vi "CHECK BATT DATA.vi"(10 "DATA":dbl[](array[numeric]), 11 "BATTERY EMULATOR":T1) -> (3 "result":bool)   [LabVIEW 2018]
panel:
  out "POWER":bool
  out "CURRENT":bool
  out "VOLTAGE":bool
  out "CONTROL SELECTED":bool
  out "MODE SELECTED":bool
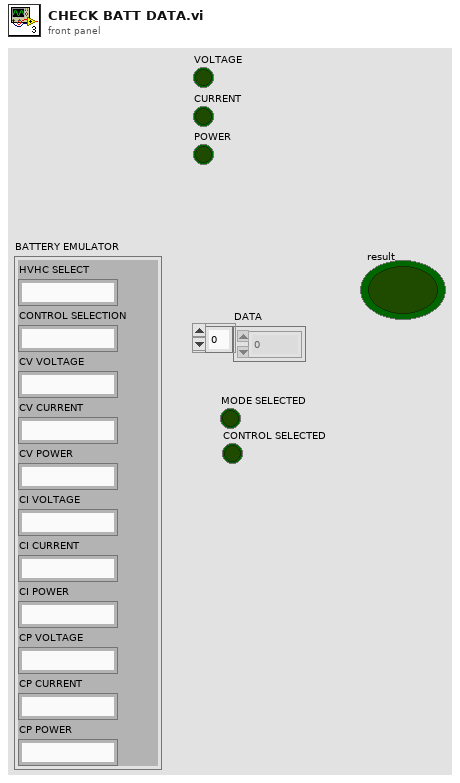
[diagram p1: front panel]
types:
  T1 = cluster{"HVHC SELECT":string, "CONTROL SELECTION":string, "CV VOLTAGE":string, "CV CURRENT":string, "CV POWER":string, "CI VOLTAGE":string, "CI CURRENT":string, "CI POWER":string, "CP VOLTAGE":string, "CP CURRENT":string, "CP POWER":string}
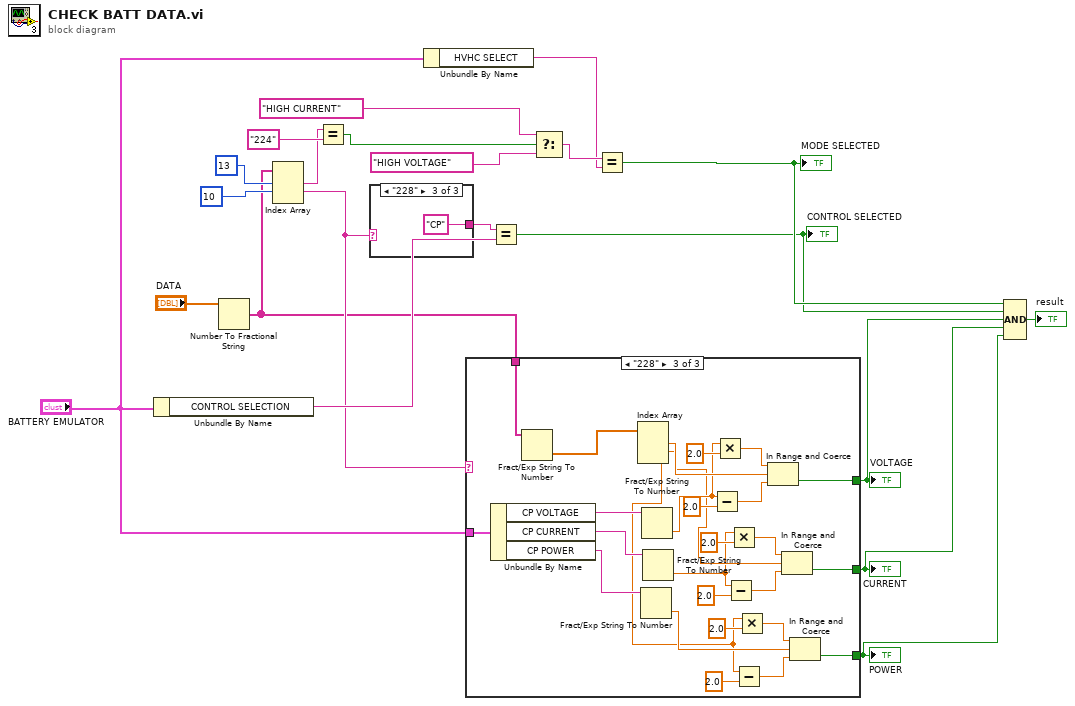
[diagram p0: block diagram]
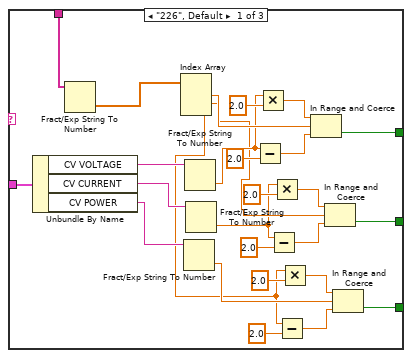
[diagram p2: hidden frame]
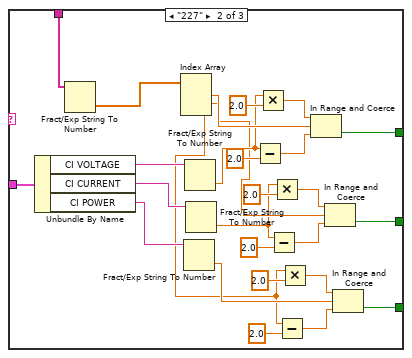
[diagram p3: hidden frame]
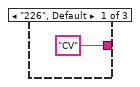
[diagram p4: hidden frame]
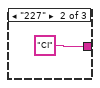
[diagram p5: hidden frame]
diagram:
  n1 = Unbundle By Name("BATTERY EMULATOR") -> ("CONTROL SELECTION"=w10:string)
  n2 = Number To Fractional String(number="DATA") -> (F-format string=w7:string[])  [unwired: 3 in]
  n3 = Index Array(array=w7, index #1=13 ("index"), index #2=10 ("index")) -> (element #1=w11:string, element #2=w9:string)  [unwired: 1 in, 1 out]
  n4 = Equal?(x=w11, y="224") -> (x = y?=w18:bool)
  n5 = case shown="\"228\"" w9 {
    tunnel: ["CV" "CI" "CP"] -> w12
    frame "226", Default {
    }
    frame "227" {
    }
    frame "228" {
    }
  }
  n6 = Unbundle By Name("BATTERY EMULATOR") -> ("HVHC SELECT"=w13:string)
  n7 = case shown="\"228\"" w9 {
    tunnel: "BATTERY EMULATOR" -> [w51 w78 w105]
    tunnel: w7 -> [w50 w77 w104]
    tunnel: [w39 w66 w93] -> w4
    tunnel: [w32 w59 w86] -> w3
    tunnel: [w26 w53 w80] -> w2
    frame "226", Default {
      n8 = Unbundle By Name(w51) -> ("CV VOLTAGE"=w48:string, "CV CURRENT"=w47:string, "CV POWER"=w46:string)
      n9 = Fract/Exp String To Number(string=w50) -> (number=w49:dbl[])  [unwired: 3 in, 1 out]
      n10 = Index Array(array=w49) -> (element #1=w45:dbl, element #2=w34:dbl, element #3=w25:dbl)  [unwired: 3 in]
      n11 = Fract/Exp String To Number(string=w46) -> (number=w27:dbl)  [unwired: 3 in, 1 out]
      n12 = Fract/Exp String To Number(string=w48) -> (number=w40:dbl)  [unwired: 3 in, 1 out]
      n13 = Fract/Exp String To Number(string=w47) -> (number=w33:dbl)  [unwired: 3 in, 1 out]
      n14 = Subtract(x=w40, y=2.0) -> (x-y=w43:dbl)
      n15 = Multiply(x=w40, y=2.0) -> (x*y=w41:dbl)
      n16 = Subtract(x=w33, y=2.0) -> (x-y=w36:dbl)
      n17 = Multiply(x=w33, y=2.0) -> (x*y=w38:dbl)
      n18 = Subtract(x=w25, y=2.0) -> (x-y=w30:dbl)
      n19 = Multiply(x=w25, y=2.0) -> (x*y=w28:dbl)
      n20 = In Range and Coerce(upper limit=w41, x=w45, lower limit=w43) -> (In Range?=w39:bool)  [unwired: 1 out]
      n21 = In Range and Coerce(upper limit=w38, x=w34, lower limit=w36) -> (In Range?=w32:bool)  [unwired: 1 out]
      n22 = In Range and Coerce(upper limit=w28, x=w27, lower limit=w30) -> (In Range?=w26:bool)  [unwired: 1 out]
    }
    frame "227" {
      n23 = Unbundle By Name(w78) -> ("CI VOLTAGE"=w75:string, "CI CURRENT"=w74:string, "CI POWER"=w73:string)
      n24 = Fract/Exp String To Number(string=w77) -> (number=w76:dbl[])  [unwired: 3 in, 1 out]
      n25 = Index Array(array=w76) -> (element #1=w72:dbl, element #2=w61:dbl, element #3=w52:dbl)  [unwired: 3 in]
      n26 = Fract/Exp String To Number(string=w73) -> (number=w54:dbl)  [unwired: 3 in, 1 out]
      n27 = Fract/Exp String To Number(string=w75) -> (number=w67:dbl)  [unwired: 3 in, 1 out]
      n28 = Fract/Exp String To Number(string=w74) -> (number=w60:dbl)  [unwired: 3 in, 1 out]
      n29 = Subtract(x=w67, y=2.0) -> (x-y=w70:dbl)
      n30 = Multiply(x=w67, y=2.0) -> (x*y=w68:dbl)
      n31 = Subtract(x=w60, y=2.0) -> (x-y=w63:dbl)
      n32 = Multiply(x=w60, y=2.0) -> (x*y=w65:dbl)
      n33 = Subtract(x=w52, y=2.0) -> (x-y=w57:dbl)
      n34 = Multiply(x=w52, y=2.0) -> (x*y=w55:dbl)
      n35 = In Range and Coerce(upper limit=w68, x=w72, lower limit=w70) -> (In Range?=w66:bool)  [unwired: 1 out]
      n36 = In Range and Coerce(upper limit=w65, x=w61, lower limit=w63) -> (In Range?=w59:bool)  [unwired: 1 out]
      n37 = In Range and Coerce(upper limit=w55, x=w54, lower limit=w57) -> (In Range?=w53:bool)  [unwired: 1 out]
    }
    frame "228" {
      n38 = Unbundle By Name(w105) -> ("CP VOLTAGE"=w102:string, "CP CURRENT"=w101:string, "CP POWER"=w100:string)
      n39 = Fract/Exp String To Number(string=w104) -> (number=w103:dbl[])  [unwired: 3 in, 1 out]
      n40 = Index Array(array=w103) -> (element #1=w99:dbl, element #2=w88:dbl, element #3=w79:dbl)  [unwired: 3 in]
      n41 = Fract/Exp String To Number(string=w100) -> (number=w81:dbl)  [unwired: 3 in, 1 out]
      n42 = Fract/Exp String To Number(string=w102) -> (number=w94:dbl)  [unwired: 3 in, 1 out]
      n43 = Fract/Exp String To Number(string=w101) -> (number=w87:dbl)  [unwired: 3 in, 1 out]
      n44 = Subtract(x=w94, y=2.0) -> (x-y=w97:dbl)
      n45 = Multiply(x=w94, y=2.0) -> (x*y=w95:dbl)
      n46 = Subtract(x=w87, y=2.0) -> (x-y=w90:dbl)
      n47 = Multiply(x=w87, y=2.0) -> (x*y=w92:dbl)
      n48 = Subtract(x=w79, y=2.0) -> (x-y=w84:dbl)
      n49 = Multiply(x=w79, y=2.0) -> (x*y=w82:dbl)
      n50 = In Range and Coerce(upper limit=w95, x=w99, lower limit=w97) -> (In Range?=w93:bool)  [unwired: 1 out]
      n51 = In Range and Coerce(upper limit=w92, x=w88, lower limit=w90) -> (In Range?=w86:bool)  [unwired: 1 out]
      n52 = In Range and Coerce(upper limit=w82, x=w81, lower limit=w84) -> (In Range?=w80:bool)  [unwired: 1 out]
    }
  }
  "VOLTAGE" <- w4
  "CURRENT" <- w3
  "POWER" <- w2
  n53 = Equal?(x=w12, y=w10) -> (x = y?=w5:bool)
  "CONTROL SELECTED" <- w5
  n54 = Select(t="HIGH CURRENT", s=w18, f="HIGH VOLTAGE") -> (s? t:f=w14:string)
  n55 = Equal?(x=w14, y=w13) -> (x = y?=w6:bool)
  "MODE SELECTED" <- w6
  n56 = Compound Arithmetic op=AND(w6, w5, w4, w3, w2) -> (→"result":bool)
